vi "Gradient Test Host Code.vi"() -> ()   [LabVIEW 2013, in "MyHostCode.lvlib"]
uses:
  MyHostCode.lvlib
  <vilib>/rvi/interface/nirviOpenFPGA/nirviOpenFPGA.xnode
  <vilib>/rvi/interface/nirviMethod/nirviMethod.xnode
  <vilib>/FPGAPlugInAG/Dynamic/niLvFpga_Reset_Dynamic.vi
  <vilib>/FPGAPlugInAG/Dynamic/niLvFpga_Run_Dynamic.vi
  <vilib>/FPGAPlugInAG/Dynamic/niLvFpga_ReadFifo_Dynamic.vi
  <vilib>/rvi/errors/niLvFpgaMergeErrorWithErrorCode.vi
  FPGA Bitfiles/ECGPWMAdaptiveFi_FPGATarget2_GradientTestFPGA_3Eq9jiaZaHM.lvbitx
  <vilib>/FPGAPlugInAG/USB-7856R/niLvFpga_Open_USB-7856R.vi
  <vilib>/rvi/interface/common/dynamic/niFpgaDynamicAddResources.vi
panel:
  out "Waveform Chart":i16[][](graph)
  in  "Stop Button":bool
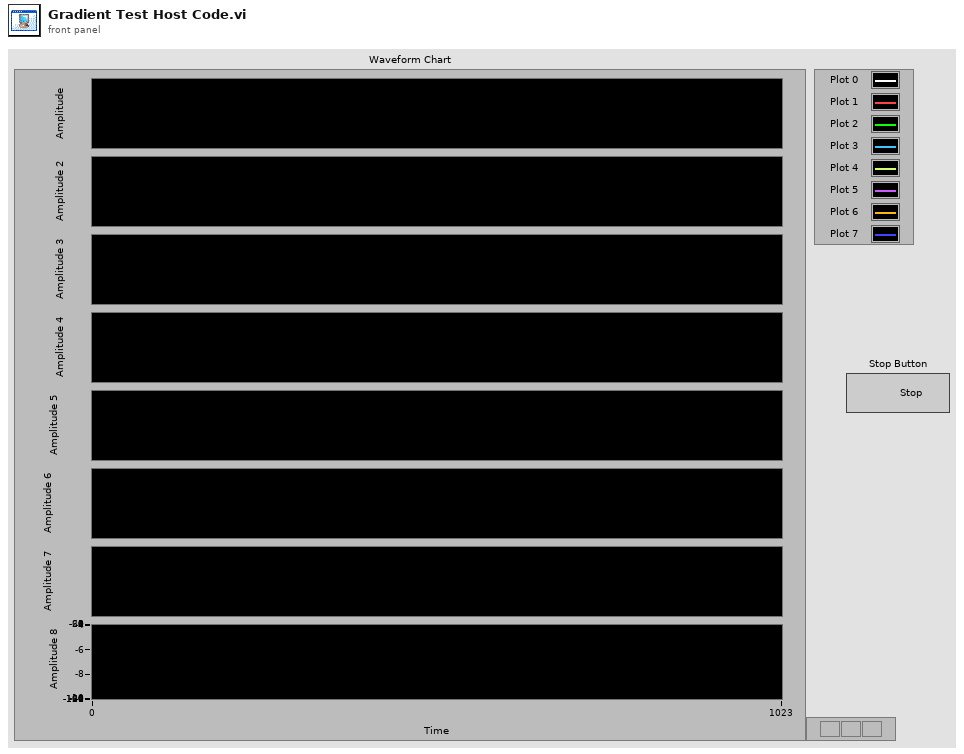
[diagram p1: front panel]
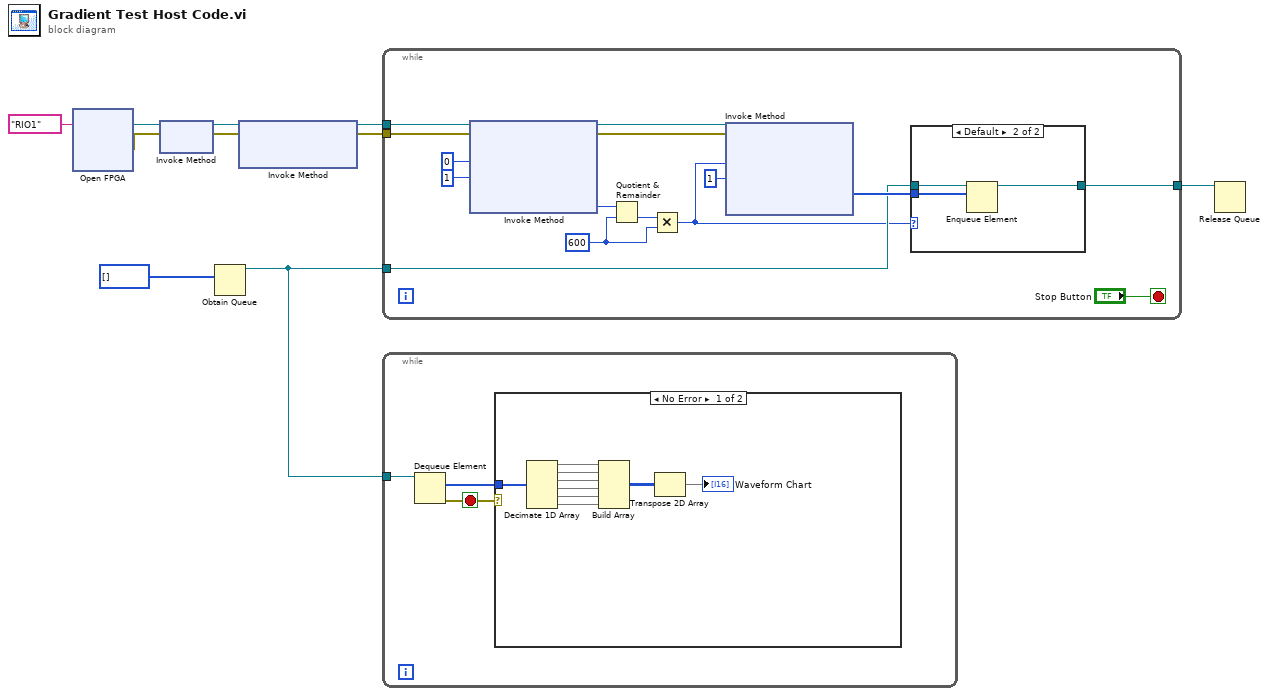
[diagram p0: block diagram]
diagram:
  n1 = xnode ("Open FPGA")("resource name"=tag "RIO1") -> ("FPGA VI Reference Out"=w9:refnum<k20>, "error out"=w8:errorcluster)  [unwired: 1 in]
  n2 = xnode ("Invoke Method")("FPGA VI Reference In"=w9, "error in"=w8) -> ("FPGA VI Reference Out"=w6:refnum<k20>, "error out"=w10:errorcluster)
  n3 = Obtain Queue(element data type=i16[] [] ("Data")) -> (queue out=w1:refnum<queue>)  [unwired: 4 in, 2 out]
  n4 = xnode ("Invoke Method")("FPGA VI Reference In"=w6, "error in"=w10) -> ("FPGA VI Reference Out"=w5:refnum<k20>, "error out"=w4:errorcluster)  [unwired: 1 in]
  n5 = while {
    tunnel: w5 -> [w25]
    tunnel: w4 -> [w24]
    tunnel: w1 -> [w13]
    tunnel: [w12] -> w2
    stop <- "Stop Button" stop-if-true
    w20 = u32 600 ("y")
    n6 = xnode ("Invoke Method")("FPGA VI Reference In"=w25, "error in"=w24, "Number of Elements"=u32 0, "Timeout (ms)"=1) -> ("FPGA VI Reference Out"=w18:refnum<k20>, "error out"=w17:errorcluster, "Elements Remaining"=w19:u32)  [unwired: 1 out]
    n7 = Quotient & Remainder(x=w19, y=w20) -> (floor(x/y)=w21:u32)  [unwired: 1 out]
    n8 = Multiply(x=w21, y=w20) -> (x*y=w11:u32)
    n9 = xnode ("Invoke Method")("FPGA VI Reference In"=w18, "error in"=w17, "Number of Elements"=w11, "Timeout (ms)"=1) -> ("Data"=w14:i16[])  [unwired: 3 out]
    n10 = case shown="Default" w11 {
      tunnel: w13 -> [w26 w29]
      tunnel: w14 -> [_ w28]
      tunnel: [w26 w27] -> w12
      frame 0 {
      }
      frame Default {
        n11 = Enqueue Element(queue=w29, element=w28) -> (queue out=w27:refnum<queue>)  [unwired: 2 in, 2 out]
      }
    }
  }
  n12 = while {
    tunnel: w1 -> [w32]
    stop <- w31 stop-if-true
    n13 = Dequeue Element(queue=w32) -> (element=w30:i16[], error out=w31:errorcluster)  [unwired: 2 in, 2 out]
    n14 = case shown="No Error" w31 {
      tunnel: w30 -> [w41 _]
      frame No Error {
        n15 = Decimate 1D Array(w41) -> (w37:i16[], w38:i16[], w39:i16[], w40:i16[], w34:i16[], w33:i16[])
        n16 = Build Array(w37, w38, w39, w40, w34, w33) -> (w36:i16[][])
        n17 = Transpose 2D Array(2D array=w36) -> (transposed array=→"Waveform Chart":i16[][])
      }
      frame Error {
      }
    }
  }
  n18 = Release Queue(queue=w2) -> ()  [unwired: 2 in, 3 out]
